vi "5790A Get Spec.vi"(8 "period":enum16{"90day", "1year", "2year"}(ring), 10 "f [Hz]":dbl, 11 "U [V]":dbl) -> (2 "rel unc(U) [ppm]":dbl, 3 "abs unc(U) [V]":dbl)   [LabVIEW 2020]
doc: "Get specification of Fluke 5790A for AC measurement assuming optimal auto range. Input 1/2 only."
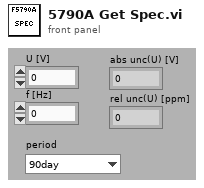
[diagram p1: front panel]
types:
  T1 = cluster{"range":dbl, "spec":cluster{"f":dbl, "90d":dbl[], "1y":dbl[], "2y":dbl[]}[]}[]
  T2 = cluster{"f":dbl, "90d":dbl[], "1y":dbl[], "2y":dbl[]}[]
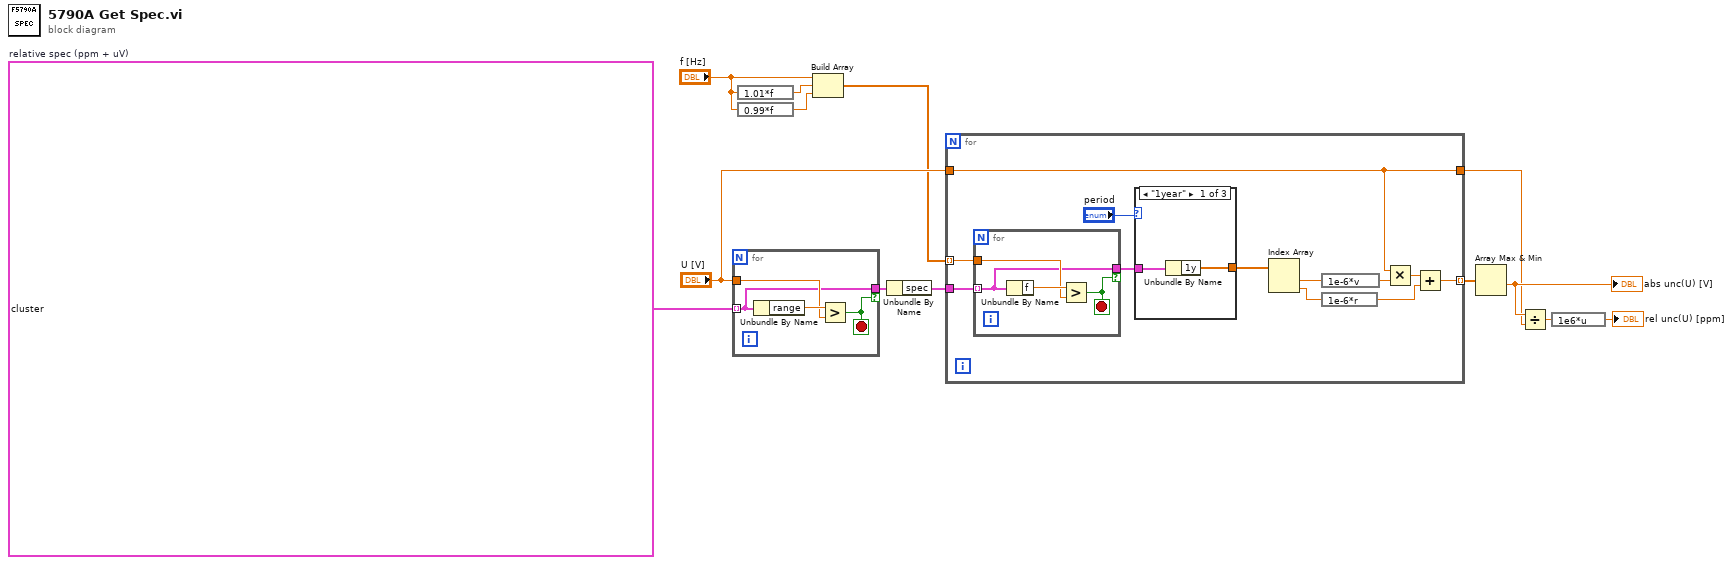
[diagram p0: block diagram]
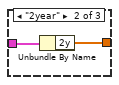
[diagram p2: hidden frame]
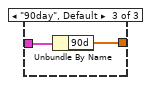
[diagram p3: hidden frame]
diagram:
  w13 = T1 [{"range"=0.0022, "spec"=[{"f"=20.0, "90d"=[100.0, 1.3], "1y"=[110.0, 1.3], "2y"=[110.0, 1.3]}, {"f"=40.0, "90d"=[54.0, 1.3], "1y"=[64.0, 1.3], "2y"=[68.0, 1.3]}, {"f"=20000.0, "90d"=[44.0, 1.3], "1y"=[59.0, 1.3], "2y"=[61.0, 1.3]}, {"f"=50000.0, "90d"=[57.0, 2.0], "1y"=[67.0, 2.0], "2y"=[110.0, 2.0]}, {"f"=100000.0, "90d"=[79.0, 2.5], "1y"=[86.0, 2.5], "2y"=[120.0, 2.5]}, {"f"=300000.0, "90d"=[190.0, 4.0], "1y"=[230.0, 4.0], "2y"=[390.0, 4.0]}, {"f"=500000.0, "90d"=[590.0, 6.0], "1y"=[720.0, 8.0], "2y"=[1200.0, 8.0]}, {"f"=1000000.0, "90d"=[2200.0, 6.0], "1y"=[2600.0, 8.0], "2y"=[4400.0, 8.0]}]}, {"range"=0.007, "spec"=[{"f"=20.0, "90d"=[80.0, 1.3], "1y"=[83.0, 1.3], "2y"=[86.0, 1.3]}, {"f"=40.0, "90d"=[33.0, 1.3], "1y"=[39.0, 1.3], "2y"=[45.0, 1.3]}, {"f"=20000.0, "90d"=[29.0, 1.3], "1y"=[36.0, 1.3], "2y"=[42.0, 1.3]}, {"f"=50000.0, "90d"=[40.0, 2.0], "1y"=[40.0, 2.0], "2y"=[63.0, 2.0]}, {"f"=100000.0, "90d"=[53.0, 2.5], "1y"=[57.0, 2.5], "2y"=[72.0, 2.5]}, {"f"=300000.0, "90d"=[110.0, 4.0], "1y"=[130.0, 4.0], "2y"=[210.0, 4.0]}, {"f"=500000.0, "90d"=[370.0, 6.0], "1y"=[450.0, 8.0], "2y"=[740.0, 8.0]}, {"f"=1000000.0, "90d"=[1600.0, 6.0], "1y"=[2000.0, 8.0], "2y"=[3400.0, 8.0]}]}, {"range"=0.022, "spec"=[{"f"=20.0, "90d"=[69.0, 1.3], "1y"=[72.0, 1.3], "2y"=[75.0, 1.3]}, {"f"=40.0, "90d"=[34.0, 1.3], "1y"=[40.0, 1.3], "2y"=[46.0, 1.3]}, {"f"=20000.0, "90d"=[30.0, 1.3], "1y"=[36.0, 1.3], "2y"=[43.0, 1.3]}, {"f"=50000.0, "90d"=[40.0, 2.0], "1y"=[45.0, 2.0], "2y"=[64.0, 2.0]}, {"f"=100000.0, "90d"=[53.0, 2.5], "1y"=[57.0, 2.5], "2y"=[73.0, 2.5]}, {"f"=300000.0, "90d"=[97.0, 4.0], "1y"=[110.0, 4.0], "2y"=[160.0, 4.0]}, {"f"=500000.0, "90d"=[310.0, 6.0], "1y"=[380.0, 8.0], "2y"=[610.0, 8.0]}, {"f"=1000000.0, "90d"=[1200.0, 6.0], "1y"=[2000.0, 8.0], "2y"=[2500.0, 8.0]}]}, {"range"=0.07, "spec"=[{"f"=20.0, "90d"=[60.0, 1.5], "1y"=[61.0, 1.5], "2y"=[62.0, 1.5]}, {"f"=40.0, "90d"=[27.0, 1.5], "1y"=[30.0, 1.5], "2y"=[37.0, 1.5]}, {"f"=20000.0, "90d"=[22.0, 1.5], "1y"=[25.0, 1.5], "2y"=[34.0, 1.5]}, {"f"=50000.0, "90d"=[34.0, 2.0], "1y"=[36.0, 2.0], "2y"=[44.0, 2.0]}, {"f"=100000.0, "90d"=[53.0, 2.5], "1y"=[54.0, 2.5], "2y"=[62.0, 2.5]}, {"f"=300000.0, "90d"=[110.0, 4.0], "1y"=[120.0, 4.0], "2y"=[170.0, 4.0]}, {"f"=500000.0, "90d"=[270.0, 6.0], "1y"=[290.0, 8.0], "2y"=[320.0, 8.0]}, {"f"=1000000.0, "90d"=[910.0, 6.0], "1y"=[1500.0, 8.0], "2y"=[2500.0, 8.0]}]}, {"range"=0.22, "spec"=[{"f"=20.0, "90d"=[60.0, 1.5], "1y"=[61.0, 1.5], "2y"=[62.0, 1.5]}, {"f"=40.0, "90d"=[27.0, 1.5], "1y"=[29.0, 1.5], "2y"=[35.0, 1.5]}, {"f"=20000.0, "90d"=[22.0, 1.5], "1y"=[24.0, 1.5], "2y"=[31.0, 1.5]}, {"f"=50000.0, "90d"=[22.0, 2.0], "1y"=[24.0, 2.0], "2y"=[33.0, 2.0]}, {"f"=100000.0, "90d"=[51.0, 2.5], "1y"=[52.0, 2.5], "2y"=[59.0, 2.5]}, {"f"=300000.0, "90d"=[100.0, 4.0], "1y"=[120.0, 4.0], "2y"=[170.0, 4.0]}, {"f"=500000.0, "90d"=[260.0, 6.0], "1y"=[290.0, 8.0], "2y"=[310.0, 8.0]}, {"f"=1000000.0, "90d"=[890.0, 6.0], "1y"=[950.0, 8.0], "2y"=[1200.0, 8.0]}]}, {"range"=0.7, "spec"=[{"f"=20.0, "90d"=[60.0, 1.5], "1y"=[61.0, 1.5000000000000002], "2y"=[62.0, 1.5000000000000002]}, {"f"=40.0, "90d"=[27.0, 1.5], "1y"=[29.0, 1.5000000000000002], "2y"=[34.0, 1.5000000000000002]}, {"f"=20000.0, "90d"=[22.0, 1.5], "1y"=[24.0, 1.5000000000000002], "2y"=[31.0, 1.5000000000000002]}, {"f"=50000.0, "90d"=[22.0, 2.0], "1y"=[24.0, 2.0], "2y"=[33.0, 2.0]}, {"f"=100000.0, "90d"=[51.0, 2.5], "1y"=[52.0, 2.5], "2y"=[59.0, 2.5]}, {"f"=300000.0, "90d"=[100.0, 4.0], "1y"=[120.0, 4.0], "2y"=[170.0, 4.0]}, {"f"=500000.0, "90d"=[260.0, 6.0], "1y"=[270.0, 8.0], "2y"=[310.0, 8.0]}, {"f"=1000000.0, "90d"=[890.0, 6.0], "1y"=[950.0, 8.0], "2y"=[1200.0, 8.0]}]}, {"range"=2.2, "spec"=[{"f"=20.0, "90d"=[60.0, 0.0], "1y"=[61.0, 0.0], "2y"=[62.0, 0.0]}, {"f"=40.0, "90d"=[26.0, 0.0], "1y"=[28.0, 0.0], "2y"=[34.0, 0.0]}, {"f"=20000.0, "90d"=[20.0, 0.0], "1y"=[22.0, 0.0], "2y"=[27.0, 0.0]}, {"f"=50000.0, "90d"=[21.0, 0.0], "1y"=[23.0, 0.0], "2y"=[33.0, 0.0]}, {"f"=100000.0, "90d"=[49.0, 0.0], "1y"=[50.0, 0.0], "2y"=[57.0, 0.0]}, {"f"=300000.0, "90d"=[92.0, 0.0], "1y"=[110.0, 0.0], "2y"=[160.0, 0.0]}, {"f"=500000.0, "90d"=[220.0, 0.0], "1y"=[230.0, 0.0], "2y"=[280.0, 0.0]}, {"f"=1000000.0, "90d"=[830.0, 0.0], "1y"=[890.0, 0.0], "2y"=[1200.0, 0.0]}]}, {"range"=7.0, "spec"=[{"f"=20.0, "90d"=[60.0, 0.0], "1y"=[61.0, 0.0], "2y"=[62.0, 0.0]}, {"f"=40.0, "90d"=[27.0, 0.0], "1y"=[29.0, 0.0], "2y"=[36.0, 0.0]}, {"f"=20000.0, "90d"=[20.0, 0.0], "1y"=[22.0, 0.0], "2y"=[27.0, 0.0]}, {"f"=50000.0, "90d"=[23.0, 0.0], "1y"=[26.0, 0.0], "2y"=[35.0, 0.0]}, {"f"=100000.0, "90d"=[62.0, 0.0], "1y"=[64.0, 0.0], "2y"=[73.0, 0.0]}, {"f"=300000.0, "90d"=[140.0, 0.0], "1y"=[150.0, 0.0], "2y"=[180.0, 0.0]}, {"f"=500000.0, "90d"=[360.0, 0.0], "1y"=[380.0, 0.0], "2y"=[450.0, 0.0]}, {"f"=1000000.0, "90d"=[1100.0, 0.0], "1y"=[1200.0, 0.0], "2y"=[1500.0, 0.0]}]}, {"range"=22.0, "spec"=[{"f"=20.0, "90d"=[60.0, 0.0], "1y"=[61.0, 0.0], "2y"=[62.0, 0.0]}, {"f"=40.0, "90d"=[28.0, 0.0], "1y"=[30.0, 0.0], "2y"=[37.0, 0.0]}, {"f"=20000.0, "90d"=[20.0, 0.0], "1y"=[22.0, 0.0], "2y"=[27.0, 0.0]}, {"f"=50000.0, "90d"=[23.0, 0.0], "1y"=[26.0, 0.0], "2y"=[35.0, 0.0]}, {"f"=100000.0, "90d"=[62.0, 0.0], "1y"=[64.0, 0.0], "2y"=[69.0, 0.0]}, {"f"=300000.0, "90d"=[140.0, 0.0], "1y"=[150.0, 0.0], "2y"=[180.0, 0.0]}, {"f"=500000.0, "90d"=[360.0, 0.0], "1y"=[380.0, 0.0], "2y"=[450.0, 0.0]}, {"f"=1000000.0, "90d"=[1100.0, 0.0], "1y"=[1200.0, 0.0], "2y"=[1500.0, 0.0]}]}, {"range"=70.0, "spec"=[{"f"=20.0, "90d"=[60.0, 0.0], "1y"=[62.0, 0.0], "2y"=[63.0, 0.0]}, {"f"=40.0, "90d"=[29.0, 0.0], "1y"=[31.0, 0.0], "2y"=[39.0, 0.0]}, {"f"=20000.0, "90d"=[23.0, 0.0], "1y"=[25.0, 0.0], "2y"=[34.0, 0.0]}, {"f"=50000.0, "90d"=[25.0, 0.0], "1y"=[27.0, 0.0], "2y"=[39.0, 0.0]}, {"f"=100000.0, "90d"=[64.0, 0.0], "1y"=[68.0, 0.0], "2y"=[85.0, 0.0]}, {"f"=300000.0, "90d"=[140.0, 0.0], "1y"=[150.0, 0.0], "2y"=[180.0, 0.0]}, {"f"=500000.0, "90d"=[370.0, 0.0], "1y"=[380.0, 0.0], "2y"=[490.0, 0.0]}, {"f"=1000000.0, "90d"=[1100.0, 0.0], "1y"=[1200.0, 0.0], "2y"=[1500.0, 0.0]}]}, {"range"=220.0, "spec"=[{"f"=20.0, "90d"=[61.0, 0.0], "1y"=[62.0, 0.0], "2y"=[64.0, 0.0]}, {"f"=40.0, "90d"=[30.0, 0.0], "1y"=[32.0, 0.0], "2y"=[40.0, 0.0]}, {"f"=20000.0, "90d"=[23.0, 0.0], "1y"=[25.0, 0.0], "2y"=[34.0, 0.0]}, {"f"=50000.0, "90d"=[30.0, 0.0], "1y"=[34.0, 0.0], "2y"=[49.0, 0.0]}, {"f"=100000.0, "90d"=[66.0, 0.0], "1y"=[69.0, 0.0], "2y"=[83.0, 0.0]}, {"f"=300000.0, "90d"=[160.0, 0.0], "1y"=[170.0, 0.0], "2y"=[220.0, 0.0]}, {"f"=500000.0, "90d"=[410.0, 0.0], "1y"=[480.0, 0.0], "2y"=[680.0, 0.0]}]}, {"range"=700.0, "spec"=[{"f"=20.0, "90d"=[62.0, 0.0], "1y"=[63.0, 0.0], "2y"=[65.0, 0.0]}, {"f"=40.0, "90d"=[31.0, 0.0], "1y"=[33.0, 0.0], "2y"=[41.0, 0.0]}, {"f"=20000.0, "90d"=[24.0, 0.0], "1y"=[25.0, 0.0], "2y"=[31.0, 0.0]}, {"f"=50000.0, "90d"=[100.0, 0.0], "1y"=[110.0, 0.0], "2y"=[140.0, 0.0]}, {"f"=100000.0, "90d"=[390.0, 0.0], "1y"=[500.0, 0.0], "2y"=[850.0, 0.0]}]}, {"range"=1001.0, "spec"=[{"f"=20.0, "90d"=[62.0, 0.0], "1y"=[63.0, 0.0], "2y"=[65.0, 0.0]}, {"f"=40.0, "90d"=[31.0, 0.0], "1y"=[33.0, 0.0], "2y"=[41.0, 0.0]}, {"f"=20000.0, "90d"=[24.0, 0.0], "1y"=[25.0, 0.0], "2y"=[31.0, 0.0]}, {"f"=50000.0, "90d"=[100.0, 0.0], "1y"=[110.0, 0.0], "2y"=[140.0, 0.0]}, {"f"=100000.0, "90d"=[390.0, 0.0], "1y"=[500.0, 0.0], "2y"=[850.0, 0.0]}]}]  # relative spec (ppm + uV)
  n1 = for {
    tunnel: w13 -> [w15] mode=indexing
    tunnel: "U [V]" -> [w16]
    tunnel: [w15] -> w12 if=w14
    stop <- w14 stop-if-true
    n2 = Unbundle By Name(w15) -> ("range"=w17:dbl)
    n3 = Greater?(x=w17, y=w16) -> (0:w14:bool)
  }
  n4 = expression code="1.01*f"("f [Hz]") -> (w9:dbl)
  n5 = expression code="0.99*f"("f [Hz]") -> (w8:dbl)
  n6 = Build Array("f [Hz]", w9, w8) -> (w6:dbl[])
  n7 = Unbundle By Name(w12) -> ("spec"=w11:T2)
  n8 = for {
    tunnel: w11 -> [w29]
    tunnel: "U [V]" -> [w18]
    tunnel: w6 -> [w20] mode=indexing
    tunnel: [w19] -> w5 mode=indexing
    tunnel: [w18] -> w3
    n9 = for {
      tunnel: w29 -> [w37] mode=indexing
      tunnel: w20 -> [w38]
      tunnel: [w37] -> w28 if=w36
      stop <- w36 stop-if-true
      n10 = Unbundle By Name(w37) -> ("f"=w39:dbl)
      n11 = Greater?(x=w39, y=w38) -> (0:w36:bool)
    }
    n12 = case shown="\"1year\"" "period" {
      tunnel: w28 -> [w31 w33 w35]
      tunnel: [w30 w32 w34] -> w26
      frame "1year" {
        n13 = Unbundle By Name(w31) -> ("1y"=w30:dbl[])
      }
      frame "2year" {
        n14 = Unbundle By Name(w33) -> ("2y"=w32:dbl[])
      }
      frame "90day", Default {
        n15 = Unbundle By Name(w35) -> ("90d"=w34:dbl[])
      }
    }
    n16 = Index Array(array=w26) -> (element #1=w25:dbl, element #2=w23:dbl)  [unwired: 2 in]
    n17 = expression code="1e-6*v"(w25) -> (w24:dbl)
    n18 = expression code="1e-6*r"(w23) -> (w21:dbl)
    n19 = Multiply(x=w18, y=w24) -> (x*y=w22:dbl)
    n20 = Add(x=w22, y=w21) -> (x+y=w19:dbl)
  }
  n21 = Array Max & Min(array=w5) -> (min value=w4:dbl)  [unwired: 3 out]
  "abs unc(U) [V]" <- w4
  n22 = Divide(x=w4, y=w3) -> (x/y=w2:dbl)
  n23 = expression code="1e6*u"(w2) -> (→"rel unc(U) [ppm]":dbl)
